vi "DIM_DIO.set bit.vi"(0 "i ref in":refnum<vi>, 2 "bitValue":bool, 3 "ms timeout (10000)":i32=10000, 5 "error in (no error)":errorcluster) -> (14 "i ref out":refnum<vi>, 17 "timed out":bool, 19 "error out":errorcluster)   [LabVIEW 2014, in "DIM_DIO.lvlib"]
doc: "Sets a bit at a digital output.\n\nLicense Agreement for this software:\n\nCopyright (C)\nGesellschaft für Schwerionenforschung, GSI\nPlanckstr. 1\n64291 Darmstadt\nGermany\n\nContact: D.Beck@gsi.de \n\nThis program is free software; you can redistribute it and/or modify it under the terms of the GNU General Public License as published by the Free Software Foundation; either version 2 of the license, or (at your option) any later version.\n\nThis program is distributed in the hope that it will be useful, but WITHOUT ANY WARRANTY; without even the implied warranty of MERCHANTABILITY or FITNESS FOR A PARTICULAR PURPOSE. See the GNU General License for more details (http://www.gnu.org).\n\nGesellschaft für Schwerionenforschung, GSI\nPlanckstr. 1, 64291 Darmstadt, Germany\nFor all questions and ideas contact: M.Richter@gsi.de, H.Brand@gsi.de or D.Beck@gsi.de.\nLast update: 17-JUN-2004"
uses:
  DIM_DIO.lvlib
  CSCore/CSApplicationBaseClasses/DigiIOBase/DigiIOBase.directionType.ctl
  CSCore/CSApplicationBaseClasses/DigiIOBase/DigiIOBase.serviceType.ctl
  CSlibraries/UtilityLib/UtilityLib.valueStatus.ctl
  CSlibraries-extern/DimLVEvent/LVDimInterface/LVDimInterface.lvlib
  CSCore/CSApplicationBaseClasses/DigiIOBase/DigiIOBase.lvlib
  CSlibraries/UtilityLib/UtilityLib.lvlib
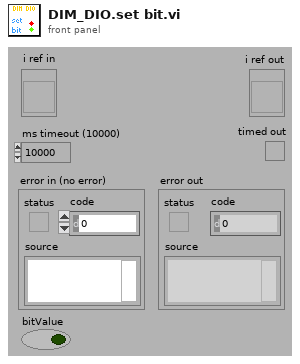
[diagram p1: front panel]
types:
  T1 = typedef "UtilityLib.lvlib/UtilityLib.valueStatus.ctl" = enum16{"no info available", "stand by/off", "on", "warning", "alarm/malfunction", "not implemented", "user action required", "important information", "system default", "control default", "indicator default", "button default"}
  T2 = typedef "DigiIOBase.lvlib/DigiIOBase.serviceType.ctl" = enum16{"bit", "word"}
  T3 = typedef "DigiIOBase.lvlib/DigiIOBase.directionType.ctl" = enum16{"unknown", "update actual value", "update nominal value", "update both"}
  T4 = typedef "DIM_DIO.lvlib/DIM_DIO.i attribute.ctl" = cluster{"serviceIDs":cluster{"writeBitID":i32}}
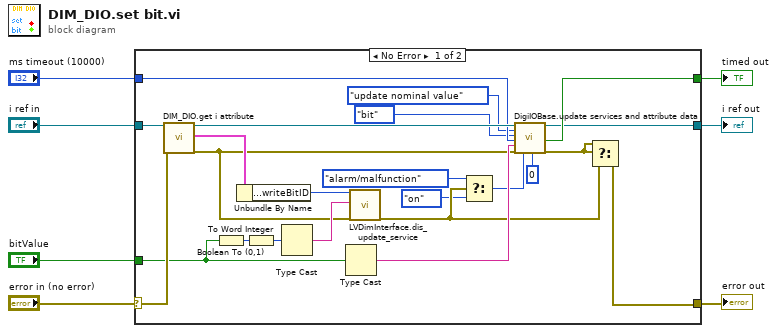
[diagram p0: block diagram]
diagram:
  n1 = case shown="No Error" "error in (no error)" {
    selector: "error in (no error)" -> [w29 w32]
    tunnel: [w14 w32] -> w6
    tunnel: "i ref in" -> [w30 w31]
    tunnel: [w8 w31] -> w4
    tunnel: "ms timeout (10000)" -> [w22 _]
    tunnel: "bitValue" -> [w18 _]
    tunnel: [w21 _] -> w1
    frame No Error {
      n2 = call "DIM_DIO.get i attribute.vi"("i ref in"=w30, "error in (no error)"=w29) -> ("i ref out"=w23:refnum<vi>, "i attribute"=w28:T4, "error out"=w16:errorcluster)  [unwired: 15 in]
      n3 = Boolean To (0,1)(Boolean=w18) -> (0, 1=w26:i16)
      n4 = Unbundle By Name(w28) -> ("serviceIDs.writeBitID"=w27:i32)
      n5 = To Word Integer(number=w26) -> (16bit integer=w25:i16)
      n6 = Type Cast(x=w25) -> (*(type *) &x=w24:string)  [unwired: 1 in]
      n7 = Type Cast(x=w18) -> (*(type *) &x=w17:string)  [unwired: 1 in]
      n8 = call "LVDimInterface.dis_update_service.vi"("my_serviceID"=w27, "data"=w24, "error in (no error)"=w16) -> ("error out"=w13:errorcluster)  [unwired: 14 in, 2 out]
      n9 = Select(t=UtilityLib.valueStatus."alarm/malfunction", s=w13, f=UtilityLib.valueStatus."on" ("quality")) -> (s? t:f=w10:T1)
      n10 = call "DigiIOBase.update services and attribute data.vi"("i ref in"=w23, "direction"=DigiIOBase.directionType."update nominal value", "service"=DigiIOBase.serviceType."bit", "ms timeout (10000)"=w22, "value"=w17, "error in (no error)"=w16, "quality"=w10, "index"=0) -> ("i ref out"=w8:refnum<vi>, "timed out"=w21:bool, "error out"=w15:errorcluster)  [unwired: 9 in]
      n11 = Select(t=w15, s=w15, f=w13) -> (s? t:f=w14:errorcluster)
    }
    frame Error {
    }
  }
  "error out" <- w6
  "i ref out" <- w4
  "timed out" <- w1
